vi "can_decoder.vi"() -> ()   [LabVIEW 2015]
panel:
  out "appended array":string[](array[string])
  out "x != y?":bool[](array[boolean])
  out "data rev 3":u64 format="%0x"
  in  "end":i32
  out "data rev 2":u64 format="%0x"
  in  "start":u16
  out "selective data":string
  in  "IDs":string
  out "data rev":u64 format="%016x"
  out "can_log":string
  in  "clear":bool
  in  "ID":i32 format="%03x"
  out "data":u64 format="%016x"
  out "error out":errorcluster
  out "Data":u8[][](array[numeric])
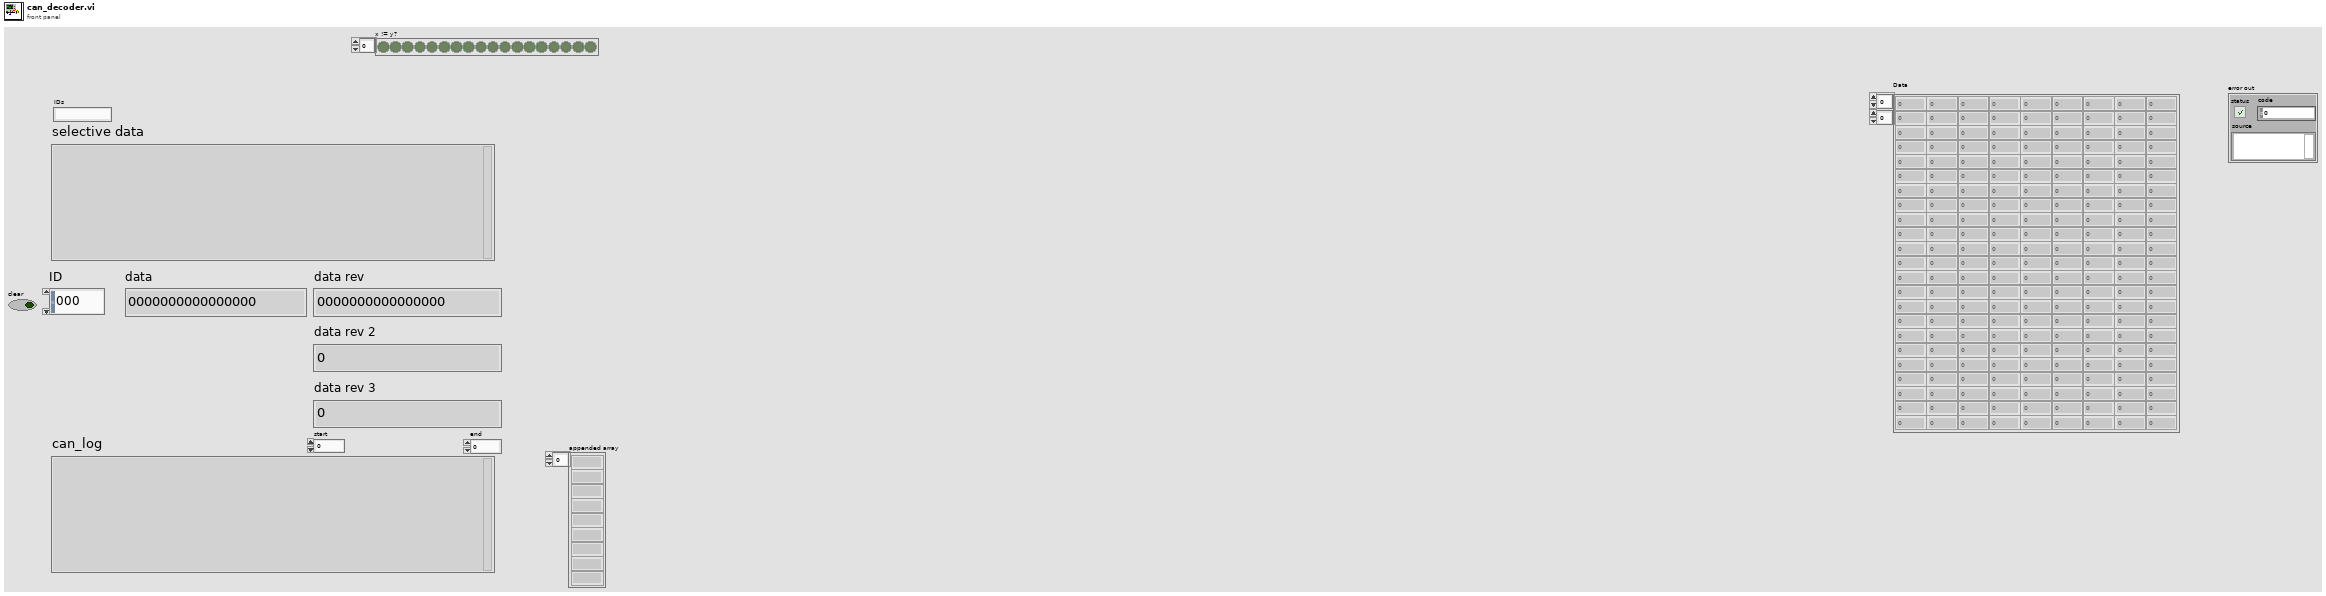
[diagram p1: front panel]
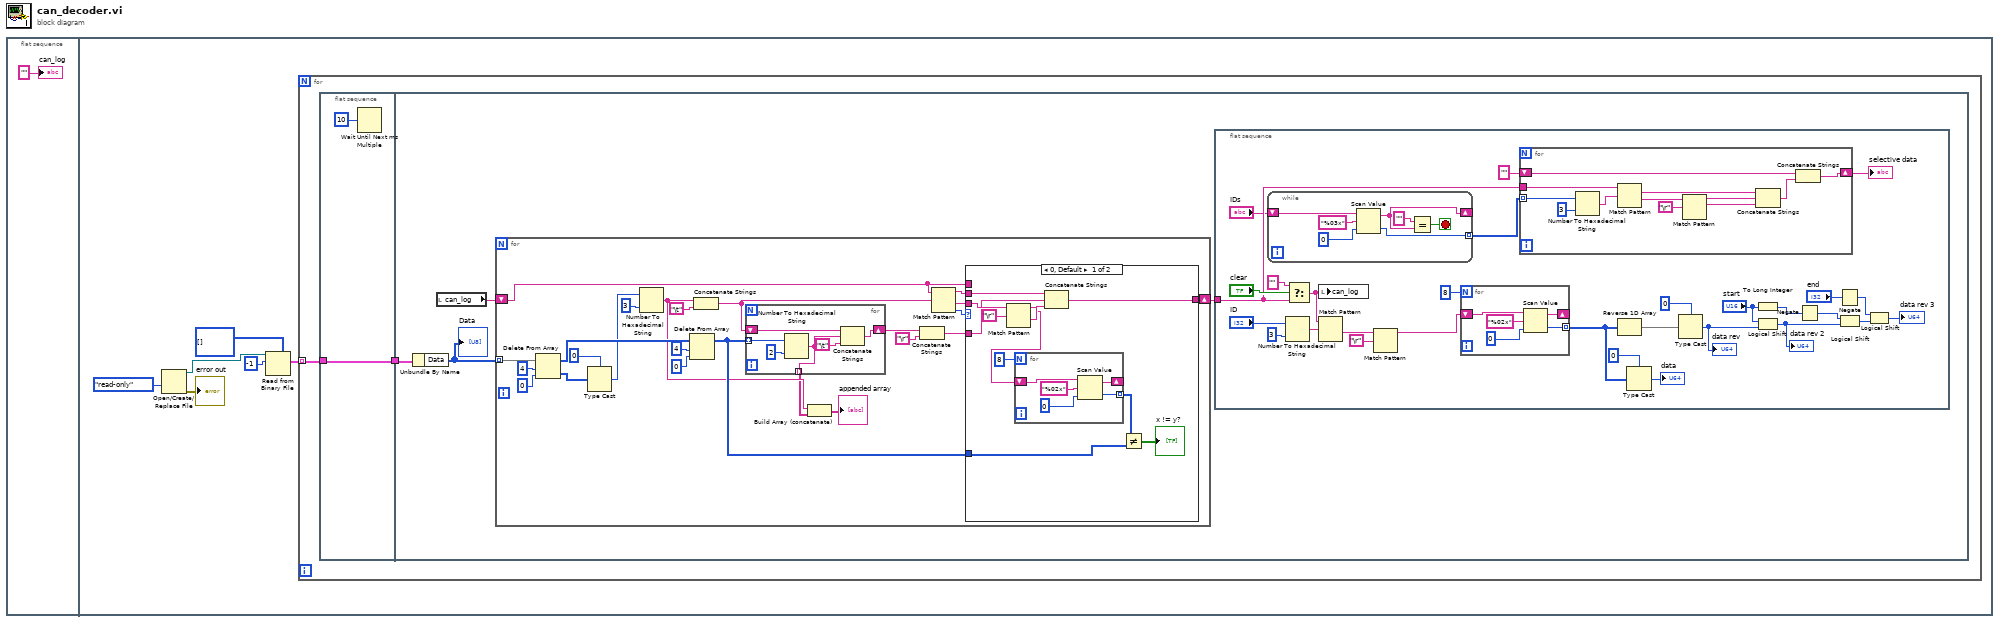
[diagram p0: block diagram]
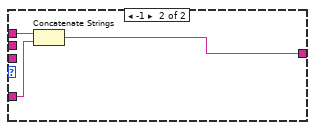
[diagram p2: hidden frame]
diagram:
  n1 = flat-sequence {
    frame #0 {
      "can_log" <- "" ("can_log")
    }
    frame #1 {
      n2 = Open/Create/Replace File(access (0:read/write)=enum16{"read/write", "read-only", "write-only"}."read-only") -> (refnum out=w2:refnum<file>, error out=→"error out":errorcluster)  [unwired: 5 in, 1 out]
      n3 = Read from Binary File(5:u8[][] [] ("Data"), 10:-1 ("count (1)"), 11:w2) -> (2:w5:cluster{"Data":u8[][]}[])  [unwired: 3 in, 3 out]
      n4 = for {
        tunnel: w5 -> [w9] mode=indexing
        n5 = flat-sequence {
          tunnel: w9 -> [w11]
          tunnel: [w11] -> w8
          tunnel: w8 -> [w15]
          frame #0 {
            n6 = Wait Until Next ms Multiple(millisecond multiple=u32 10) -> ()  [unwired: 1 out]
          }
          frame #1 {
            n7 = Unbundle By Name(w15) -> ("Data"=w12:u8[][])
            "Data" <- w12
            n8 = local read "can_log"() -> (w14:string)
            n9 = for {
              tunnel: w12 -> [w92] mode=indexing
              shift-right: [w74] -> w13
              shift-left: w14 -> [w73]
              n10 = Delete From Array(array=w92, length=4, index=0) -> (deleted portion=w89:u8[], array with subset deleted=w87:u8[])
              n11 = Type Cast(type=u32 0, x=w89) -> (*(type *) &x=w84:u32)
              n12 = Number To Hexadecimal String(1:i16 3 ("width (-)"), 2:w84) -> (0:w71:string)
              n13 = Delete From Array(array=w87, length=4, index=0) -> (array with subset deleted=w72:u8[])  [unwired: 1 out]
              n14 = Concatenate Strings(w71, "\t") -> (w79:string)
              n15 = for {
                tunnel: w72 -> [w117] mode=indexing
                shift-right: [w115] -> w83
                shift-left: w79 -> [w116]
                tunnel: [w112] -> w70 mode=indexing
                n16 = Number To Hexadecimal String(1:i16 2 ("width (-)"), 2:w117) -> (0:w112:string)
                n17 = Concatenate Strings(w116, w112, "\t") -> (w115:string)
              }
              n18 = Build Array (concatenate)(w71, w70) -> (→"appended array":string[])
              n19 = Concatenate Strings(w83, "\r") -> (w80:string)
              n20 = Match Pattern(string=w73, regular expression=w79) -> (before substring=w77:string, after substring=w76:string, offset past match=w81:i32)  [unwired: 1 in, 1 out]
              n21 = case shown="0, Default" w81 {
                tunnel: w80 -> [w99 w111]
                tunnel: w77 -> [w98 _]
                tunnel: w76 -> [w103 _]
                tunnel: [w100 w110] -> w74
                tunnel: w73 -> [_ w109]
                tunnel: w72 -> [w94 _]
                frame 0, Default {
                  n22 = Match Pattern(string=w103, regular expression="\r") -> (before substring=w96:string, after substring=w101:string)  [unwired: 1 in, 2 out]
                  n23 = for {
                    N: 8 -> [_]
                    tunnel: [w105] -> w95 mode=indexing
                    shift-right: [w104] -> _
                    shift-left: w96 -> [w108]
                    n24 = Scan Value(string=w108, format string="%02x", default (0 dbl)=u8 0 ("default (0 U32)")) -> (output string=w104:string, value=w105:u8)
                  }
                  n25 = Concatenate Strings(w98, w99, w101) -> (w100:string)
                  n26 = Not Equal?(x=w95, y=w94) -> (x != y?=→"x != y?":bool[])
                }
                frame -1 {
                  n27 = Concatenate Strings(w109, w111) -> (w110:string)
                }
              }
            }
            n28 = flat-sequence {
              tunnel: w13 -> [w29]
              frame #0 {
                n29 = while {
                  tunnel: [w48] -> w27 mode=indexing
                  shift-right: [w47] -> _
                  shift-left: "IDs" -> [w51]
                  stop <- w45 stop-if-true
                  n30 = Scan Value(string=w51, format string="%03x", default (0 dbl)=0 ("default (0 U32)")) -> (output string=w47:string, value=w48:i32)
                  n31 = Equal?(x="", y=w47) -> (x = y?=w45:bool)
                }
                n32 = Number To Hexadecimal String(1:i16 3 ("width (-)"), 2:"ID") -> (0:w40:string)
                n33 = Select(t="", s="clear", f=w29) -> (s? t:f=w42:string)
                n34 = local write "can_log"(w42) -> ()
                n35 = Match Pattern(string=w42, regular expression=w40) -> (after substring=w38:string)  [unwired: 1 in, 3 out]
                n36 = Match Pattern(string=w38, regular expression="\r") -> (before substring=w37:string)  [unwired: 1 in, 3 out]
                n37 = for {
                  N: 8 -> [_]
                  tunnel: [w65] -> w33 mode=indexing
                  shift-right: [w64] -> _
                  shift-left: w37 -> [w68]
                  n38 = Scan Value(string=w68, format string="%02x", default (0 dbl)=u8 0 ("default (0 U32)")) -> (output string=w64:string, value=w65:u8)
                }
                n39 = for {
                  tunnel: w27 -> [w62] mode=indexing
                  tunnel: w29 -> [w61]
                  shift-right: [w52] -> w25
                  shift-left: "" -> [w54]
                  n40 = Number To Hexadecimal String(1:i16 3 ("width (-)"), 2:w62) -> (0:w60:string)
                  n41 = Match Pattern(string=w61, regular expression=w60) -> (match substring=w55:string, after substring=w58:string)  [unwired: 1 in, 2 out]
                  n42 = Match Pattern(string=w58, regular expression="\r") -> (before substring=w56:string, match substring=w57:string)  [unwired: 1 in, 2 out]
                  n43 = Concatenate Strings(w55, w56, w57) -> (w53:string)
                  n44 = Concatenate Strings(w54, w53) -> (w52:string)
                }
                "selective data" <- w25
                n45 = Reverse 1D Array(array=w33) -> (reversed array=w31:u8[])
                n46 = Type Cast(type=u64 0, x=w33) -> (*(type *) &x=→"data":u64)
                n47 = Type Cast(type=u64 0, x=w31) -> (*(type *) &x=w24:u64)
                "data rev" <- w24
                n48 = To Long Integer(number="start") -> (32bit integer=w22:i32)
                n49 = Logical Shift(y="start", x=w24) -> (x << y=w17:u64)
                "data rev 2" <- w17
                n50 = Negate(x=w22) -> (-x=w21:i32)
                n51 = Negate(x="end") -> (-x=w18:i32)
                n52 = Logical Shift(y=w21, x=w17) -> (x << y=w20:u64)
                n53 = Logical Shift(y=w18, x=w20) -> (x << y=→"data rev 3":u64)
              }
            }
          }
        }
      }
    }
  }
